vi "(Sub) Qu_HVPS_3.vi"(7 "State":T2(ring), 8 "error in (no error)":errorcluster caption="에러 입력(에러 없음)", 10 "State":T1(ring)) -> (0 "error out":errorcluster caption="에러 출력", 3 "queue out":refnum<queue>)   [LabVIEW 2017]
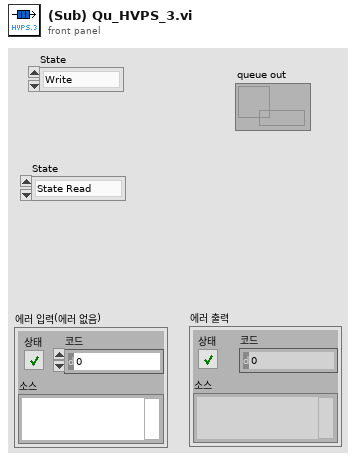
[diagram p1: front panel]
types:
  T1 = enum16{"State Read", "Data Read", "Stop", "Close"}
  T2 = enum16{"Write", "Create", "Read", "Stop", "Close"}
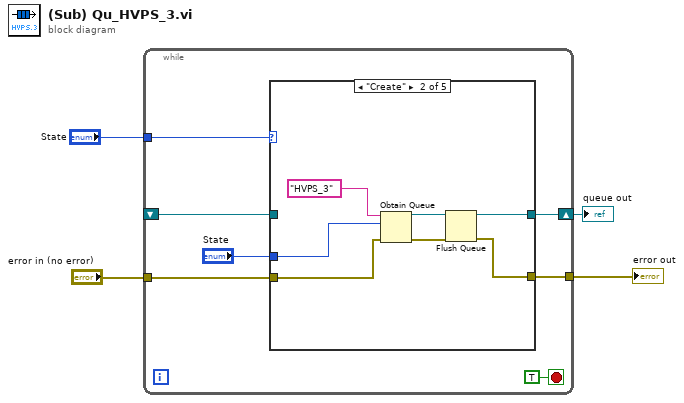
[diagram p0: block diagram]
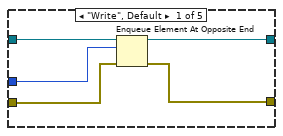
[diagram p2: hidden frame]
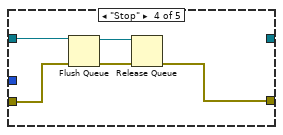
[diagram p4: hidden frame]
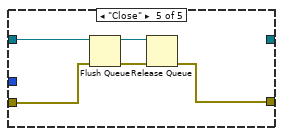
[diagram p5: hidden frame]
diagram:
  n1 = while {
    tunnel: "error in (no error)" -> [w9]
    tunnel: "State" -> [w10]
    tunnel: [w8] -> w2
    shift-right: [w7] -> w1
    shift-left: _ -> [w6]
    stop <- TRUE stop-if-true
    n2 = case shown="\"Create\"" w10 {
      tunnel: w9 -> [w14 w22 w24 w29 w34]
      tunnel: [w13 w20 w24 w26 w31] -> w8
      tunnel: "State" -> [w12 w18 _ _ _]
      tunnel: [w15 w17 w25 _ _] -> w7
      tunnel: w6 -> [w16 _ w25 w30 w35]
      frame "Write", Default {
        n3 = Enqueue Element At Opposite End(queue=w16, element=w12, error in (no error)=w14) -> (queue out=w15:refnum<queue>, error out=w13:errorcluster)  [unwired: 1 in, 1 out]
      }
      frame "Create" {
        n4 = Obtain Queue(name (unnamed)="HVPS_3" ("이름(이름없음)"), element data type=w18, error in (no error)=w22) -> (queue out=w19:refnum<queue>, error out=w21:errorcluster)  [unwired: 2 in, 1 out]
        n5 = Flush Queue(queue=w19, error in (no error)=w21) -> (queue out=w17:refnum<queue>, error out=w20:errorcluster)  [unwired: 1 out]
      }
      frame "Read" {
      }
      frame "Stop" {
        n6 = Flush Queue(queue=w30, error in (no error)=w29) -> (queue out=w27:refnum<queue>, error out=w28:errorcluster)  [unwired: 1 out]
        n7 = Release Queue(queue=w27, error in (no error)=w28) -> (error out=w26:errorcluster)  [unwired: 1 in, 2 out]
      }
      frame "Close" {
        n8 = Flush Queue(queue=w35, error in (no error)=w34) -> (queue out=w33:refnum<queue>, error out=w32:errorcluster)  [unwired: 1 out]
        n9 = Release Queue(queue=w33, error in (no error)=w32) -> (error out=w31:errorcluster)  [unwired: 1 in, 2 out]
      }
    }
  }
  "error out" <- w2
  "queue out" <- w1
